vi "CameraVision_Demo_Legacy.vi"() -> (4 "图像时间戳":u32=16532020 format="%_32g")   [LabVIEW 2015]
uses:
  MVCAMSDK.dll
  <vilib>/Analysis/NI_AALBase.lvlib
panel:
  out "variance":dbl caption="方差" format="%0.2f"
  out "相机图像":T1(plugin-control)
  out "光强图":u8[](graph)
  in  "自定义分辨率设置":bool
  in  "预设分辨率设置":bool
  out "帧速":u32
  out "帧间耗时\n单位：（0.1ms）":u32
  in  "相机枚举":T2(ring)
  in  "自动曝光模式":bool=TRUE caption="软触发"
  in  "手动曝光模式":bool caption="软触发"
  in  "硬触发模式":bool caption="软触发"
  in  "软触发模式":bool caption="软触发"
  in  "连续模式":bool caption="软触发"
  in  "软触发一帧":bool caption="软触发"
  in  "读取自定义数据":bool
  in  "写入自定义数据":bool
  in  "拍照":bool
  in  "相机参数":bool=TRUE
  in  "Stop":bool
  in  "激活预览":bool=TRUE
  out "Image":T1(plugin-control)
  # "写入自定义数据"
  # "相机原生分辨率设置"
  # "触发设置"
  # "曝光设置"
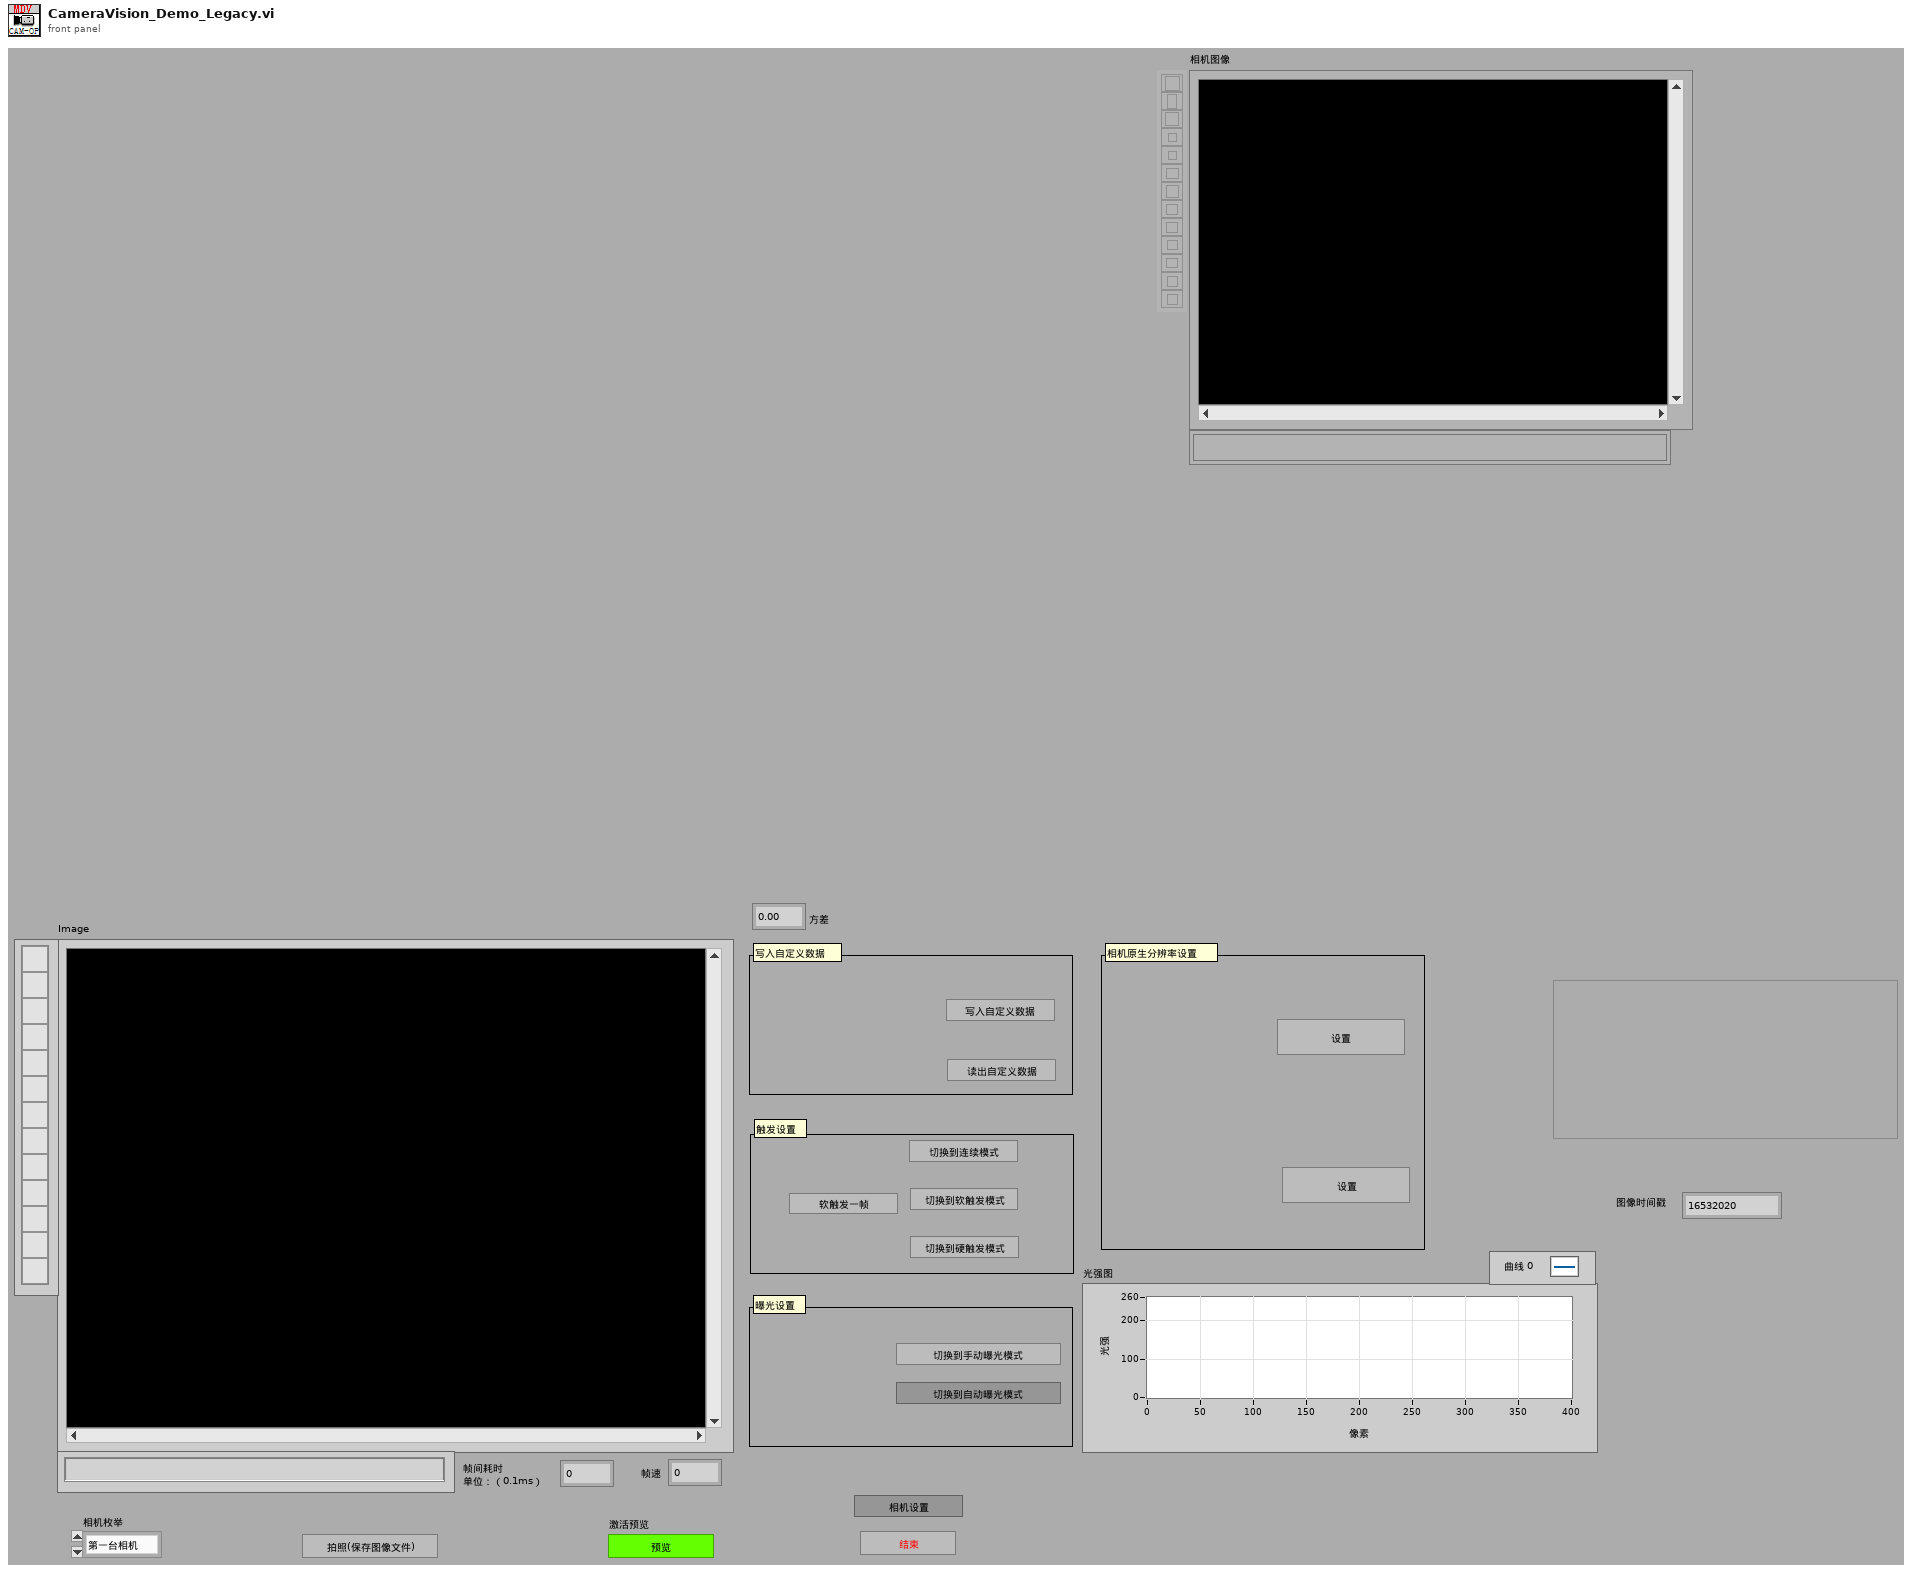
[diagram p1: front panel]
types:
  T1 = typedef "IMAQ Image.ctl" = refnum<image>
  T2 = enum16{"第一台相机", "第二台相机", "第三台相机", "第四台相机", "第五台相机"}
  T3 = typedef "Image Type" = u32
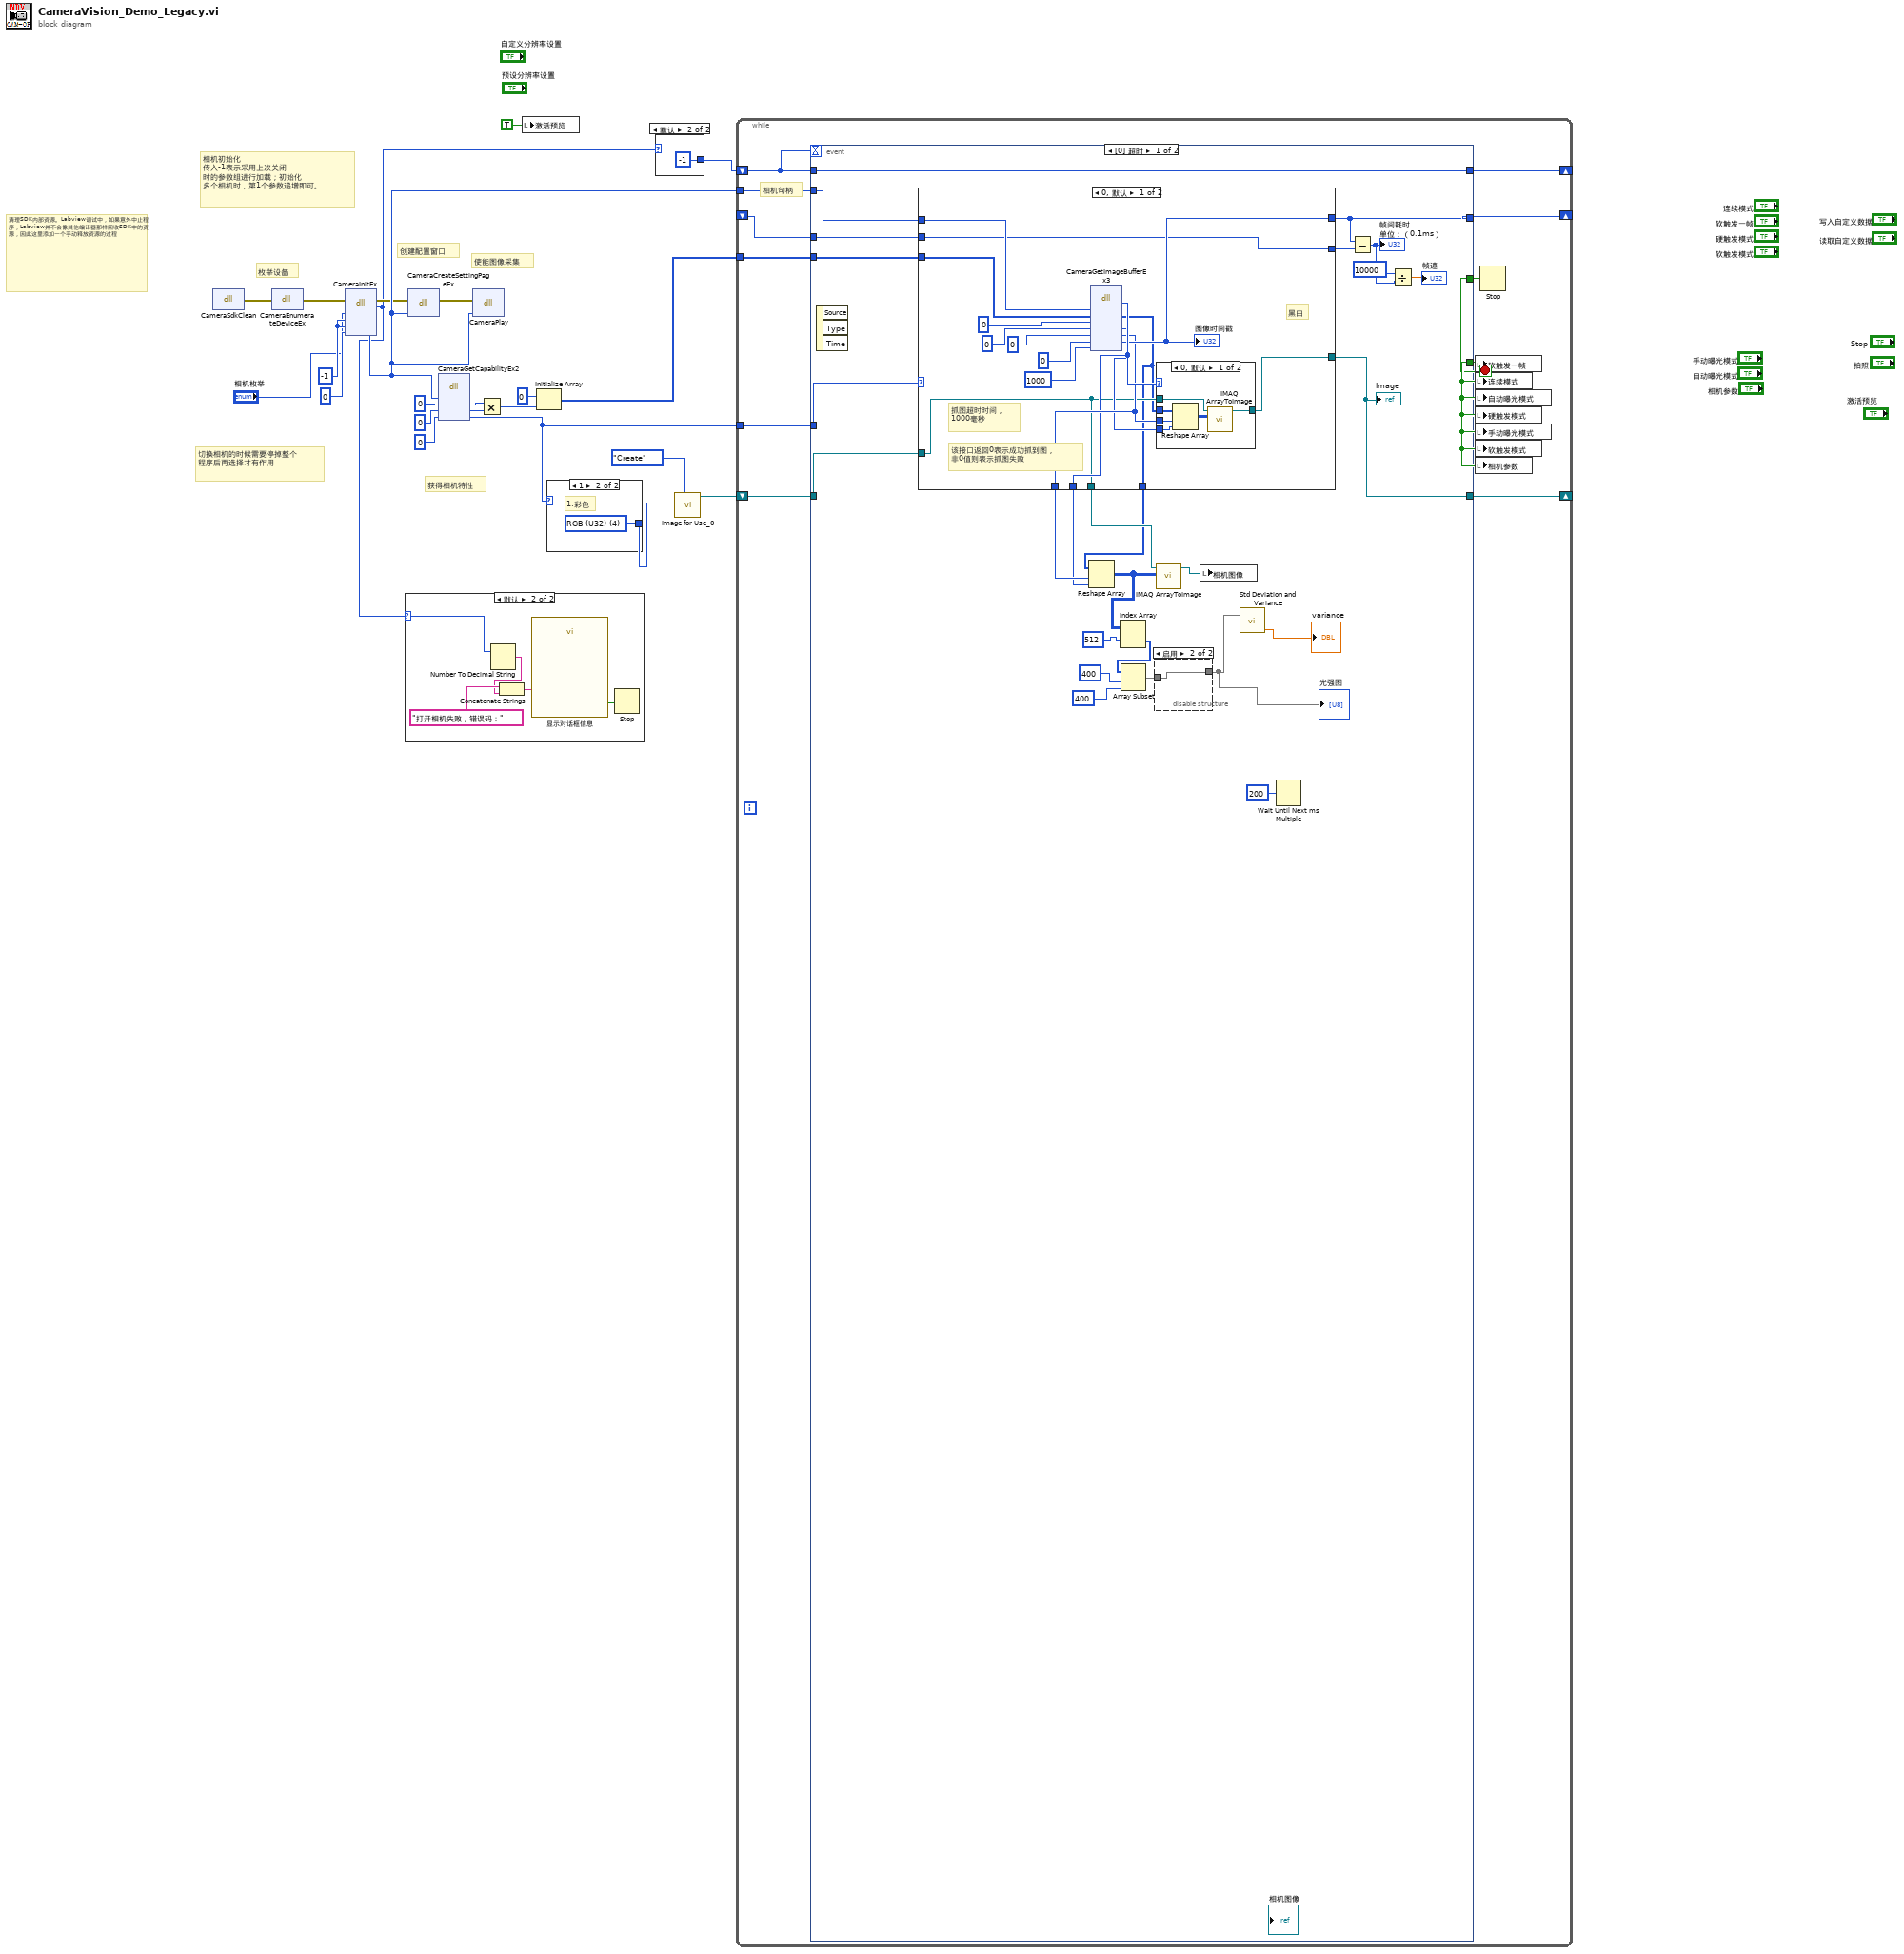
[diagram p0: block diagram]
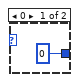
[diagram p2: hidden frame]
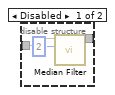
[diagram p4: hidden frame]
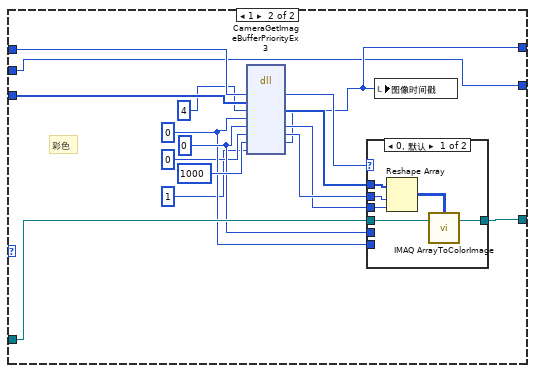
[diagram p6: hidden frame]
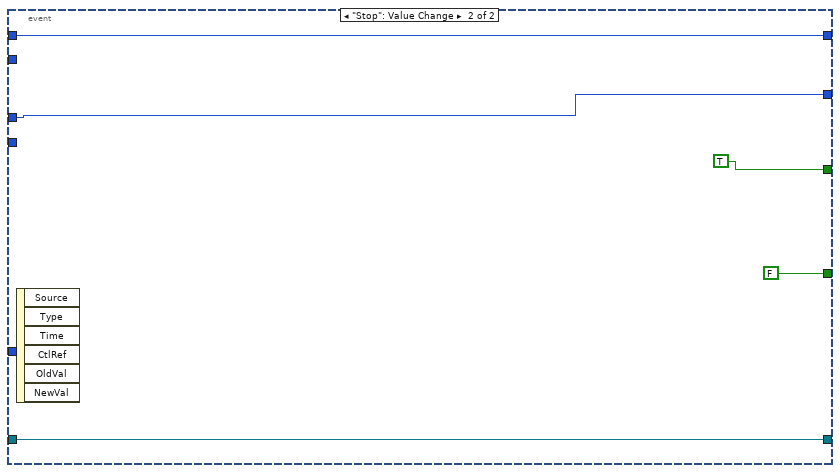
[diagram p8: hidden frame]
diagram:
  w20 = -1
  # "切换相机的时候需要停掉整个\n程序后再选择才有作用"
  # "清理SDK内部资源。Labview调试中，如果意外中止程序，Labview并不会像其他编译器那样回收SDK中的资源，因此这里添加一个手动释放资源的过程"
  # "使能图像采集"
  # "获得相机特性"
  # "创建配置窗口"
  # "相机初始化\n传入-1表示采用上次关闭\n时的参数组进行加载；初始化\n多个相机时，第1个参数递增即可。"
  # "枚举设备"
  n1 = dll-call lib="MVCAMSDK.dll" fn="CameraSdkClean"() -> (error out=w21:errorcluster)  [unwired: 4 in, 1 out]
  n2 = dll-call lib="MVCAMSDK.dll" fn="CameraEnumerateDeviceEx"(error in=w21) -> (error out=w18:errorcluster)  [unwired: 3 in, 1 out]
  n3 = dll-call lib="MVCAMSDK.dll" fn="CameraInitEx"(error in=w18, "相机索引值"="相机枚举", "参数加载方式"=w20, "要加载的参数组索引"=w20, "相机句柄"=0) -> (error out=w7:errorcluster, "返回类型"=w2:i32, "相机句柄"=w9:i32)  [unwired: 5 in, 1 out]
  n4 = case shown="默认" w2 {
    selector: w2 -> [_ w27]
    frame 0 {
    }
    frame Default {
      n5 = Number To Decimal String(number=w27) -> (decimal integer string=w24:string)  [unwired: 1 in]
      n6 = Concatenate Strings("打开相机失败，错误码：" ("字符串"), w24) -> (w26:string)
      n7 = call "显示对话框信息"("Message"=w26) -> ("结束"=w28:bool)  [unwired: 9 in, 1 out]
      n8 = Stop(stop? (T)=w28) -> ()
    }
  }
  n9 = dll-call lib="MVCAMSDK.dll" fn="CameraCreateSettingPageEx"(error in=w7, "相机句柄"=w9) -> (error out=w10:errorcluster)  [unwired: 4 in, 1 out]
  n10 = dll-call lib="MVCAMSDK.dll" fn="CameraGetCapabilityEx2"("相机句柄"=w9, "图像最大宽度"=0, "图像最大高度"=0, "是否是彩色相机(返回0:黑白;1:彩色)"=0) -> ("图像最大宽度"=w12:i32, "图像最大高度"=w11:i32, "是否是彩色相机(返回0:黑白;1:彩色)"=w6:i32)  [unwired: 5 in, 2 out]
  n11 = dll-call lib="MVCAMSDK.dll" fn="CameraPlay"(error in=w10, "相机句柄"=w9) -> ()  [unwired: 4 in, 2 out]
  n12 = Multiply(x=w12, y=w11) -> (x*y=w16:i32)
  n13 = local write "激活预览"(TRUE ("激活预览")) -> ()
  n14 = Initialize Array(0, w16) -> (w8:i32[])
  n15 = case shown="1" w6 {
    tunnel: [_ w29] -> w22
    frame 0, Default {
      # "0:黑白;"
    }
    frame 1 {
      w29 = T3 4 items=["Grayscale (U8)", "Grayscale (I16)", "Grayscale (SGL)", "Complex (CSG)", "RGB (U32)", "HSL (U32)", "RGB (U64)", "Grayscale (U16)"] ("Image Type")
      # "1:彩色"
    }
  }
  n16 = case shown="默认" w2 {
    tunnel: [0 -1] -> w1
    frame 0 {
    }
    frame Default {
    }
  }
  n17 = call "Image for Use_0.vi"("Command"=enum16{"Create", "Use", "Copy in", "Dispose"}."Create", "Image Type"=w22) -> ("Image out"=w5:T1)  [unwired: 8 in, 1 out]
  n18 = while {
    tunnel: w9 -> [w39]
    tunnel: w8 -> [w41]
    tunnel: w6 -> [w42]
    shift-right: [w38] -> _
    shift-left: w1 -> [w37]
    shift-right: [w35] -> _
    shift-left: w5 -> [w40]
    shift-right: [w34] -> _
    shift-left: _ -> [w33]
    stop <- w32 stop-if-true
    # "相机句柄"
    n19 = event shown="[0] 超时" {
      selector: _ -> [_ _]
      dyn-events: _ -> [_ _]
      timeout: w37 -> [_ _]
      tunnel: [_ TRUE] -> w32
      tunnel: w41 -> [w67 _]
      tunnel: w42 -> [w66 _]
      tunnel: w39 -> [w68 _]
      tunnel: w40 -> [w65 w119]
      tunnel: [w64 w121] -> w38
      tunnel: w37 -> [w64 w121]
      tunnel: [_ FALSE] -> w36
      tunnel: [w63 w119] -> w35
      tunnel: [w60 w118] -> w34
      tunnel: w33 -> [w62 w118]
      event Timeout {
        n20 = event-data() -> ()  [unwired: 1 in, 3 out]
        n21 = case shown="0, 默认" w66 {
          tunnel: w67 -> [w87 w110]
          tunnel: w65 -> [w74 w109]
          tunnel: w68 -> [w79 w108]
          tunnel: [w80 w98] -> w63
          tunnel: [w78 w97] -> w60
          tunnel: w62 -> [w77 w96]
          tunnel: [w77 w96] -> w61
          tunnel: [w76 _] -> w48
          tunnel: [w75 _] -> w47
          tunnel: [w74 _] -> w46
          tunnel: [w73 _] -> w45
          frame 0, Default {
            # "黑白"
            # "该接口返回0表示成功抓到图，\n非0值则表示抓图失败"
            # "抓图超时时间，\n1000毫秒"
            n22 = dll-call lib="MVCAMSDK.dll" fn="CameraGetImageBufferEx3"("相机句柄"=w79, "图像数据缓冲区"=w87, "图像输出格式(0:8位灰度;1:24位彩色;2:32位彩色，3：BGR24彩色 4：BGRA32位彩色)"=0, "图像宽度"=0, "图像高度"=0, "时间戳(单位为100微秒)"=0, "抓图超时时间(毫秒)"=1000) -> ("返回类型"=w82:i32, "图像数据缓冲区"=w73:u8[], "图像宽度"=w75:i32, "图像高度"=w76:i32, "时间戳(单位为100微秒)"=w78:u32)  [unwired: 6 in, 2 out]
            "图像时间戳" <- w78
            n23 = case shown="0, 默认" w82 {
              tunnel: w73 -> [w93 _]
              tunnel: w74 -> [w90 w94]
              tunnel: w76 -> [w92 _]
              tunnel: w75 -> [w91 _]
              tunnel: [w88 w94] -> w80
              frame 0, Default {
                n24 = Reshape Array(w93, w92, w91) -> (w89:u8[][])
                n25 = call "IMAQ ArrayToImage"("Image Pixels (U8)"=w89, "Image"=w90) -> ("Image Out"=w88:T1)  [unwired: 8 in, 1 out]
              }
              frame -12 {
              }
            }
          }
          frame 1 {
            w100 = 0
            w101 = 0
            # "彩色"
            n26 = dll-call lib="MVCAMSDK.dll" fn="CameraGetImageBufferPriorityEx3"("相机句柄"=w108, "图像数据缓冲区"=w110, "图像输出格式(0:8位灰度;1:24位彩色;2:32位彩色)"=4, "图像宽度"=w100, "图像高度"=w101, "时间戳（单位为100微秒）"=0, "抓图超时时间(毫秒)"=1000, "取图优先级(0: 取最旧   1:取最新)"=1) -> ("返回类型"=w102:i32, "图像数据缓冲区"=w105:u32[], "图像宽度"=w103:i32, "图像高度"=w104:i32, "时间戳（单位为100微秒）"=w97:u32)  [unwired: 7 in, 2 out]
            n27 = case shown="0, 默认" w102 {
              tunnel: w105 -> [w115 _]
              tunnel: w109 -> [w114 w117]
              tunnel: w104 -> [w113 _]
              tunnel: w103 -> [w112 _]
              tunnel: w101 -> [_ _]
              tunnel: w100 -> [_ _]
              tunnel: [w111 w117] -> w98
              frame 0, Default {
                n28 = Reshape Array(w115, w113, w112) -> (w116:u32[][])
                n29 = call "IMAQ ArrayToColorImage"("Image Pixels (U32)"=w116, "Image"=w114) -> ("Image Out"=w111:T1)  [unwired: 3 in, 1 out]
              }
              frame -12 {
              }
            }
            n30 = local write "图像时间戳"(w97) -> ()
          }
        }
        "Image" <- w63
        n31 = Reshape Array(w45, w48, w47) -> (w44:u8[][])
        n32 = Index Array(array=w44, index (row)=512 ("索引 (行)")) -> (element=w51:u8[])  [unwired: 1 in]
        n33 = Array Subset(array=w51, index=400 ("索引"), length=400 ("长度")) -> (w53:u8[])
        n34 = disable-structure shown="启用" {
          disable-tunnel: w53 -> [w71 w72]
          disable-tunnel: [w69 w72] -> w56
          frame Disabled {
            n35 = call <vilib>:"Median Filter.vi"("left rank"=2, "X"=w71) -> ("Filtered X"=w69:dbl[])  [unwired: 8 in, 1 out]
          }
          frame Enabled {
          }
        }
        "光强图" <- w56
        n36 = call "IMAQ ArrayToImage"("Image Pixels (U8)"=w44, "Image"=w46) -> ("Image Out"=w49:T1)  [unwired: 8 in, 1 out]
        n37 = local write "相机图像"(w49) -> ()
        n38 = call <vilib>:"Std Deviation and Variance.vi"("X"=w56) -> ("variance"=→"variance":dbl)  [unwired: 1 in, 2 out]
        n39 = Wait Until Next ms Multiple(millisecond multiple=u32 200 ("毫秒倍数")) -> ()  [unwired: 1 out]
        n40 = Subtract(x=w60, y=w61) -> (x-y=w59:u32)
        "帧间耗时\n单位：（0.1ms）" <- w59
        n41 = Divide(x=u32 10000 ("帧间耗时"), y=w59) -> (x/y=→"帧速":dbl)
      }
      event "Stop": Value Change {
        n42 = event-data() -> ()  [unwired: 1 in, 6 out]
      }
    }
    n43 = local write "软触发一帧"(w36) -> ()
    n44 = local write "连续模式"(w36) -> ()
    n45 = local write "自动曝光模式"(w36) -> ()
    n46 = local write "硬触发模式"(w36) -> ()
    n47 = local write "手动曝光模式"(w36) -> ()
    n48 = local write "软触发模式"(w36) -> ()
    n49 = local write "相机参数"(w36) -> ()
    n50 = Stop(stop? (T)=w32) -> ()
  }
